vi "Global LV.vi"() -> ()   [LabVIEW 2023, in "GUI.lvlib"]
uses:
  GUI.lvlib
panel:
  out "Uniquestepld & Result Status":variant
  in  "TestCase Status":string[](array[string])
  in  "Fail Count":i32
  in  "Pass Count":i32
  out "Interlock Started?":bool
  in  "TestCase":string[](array[string])
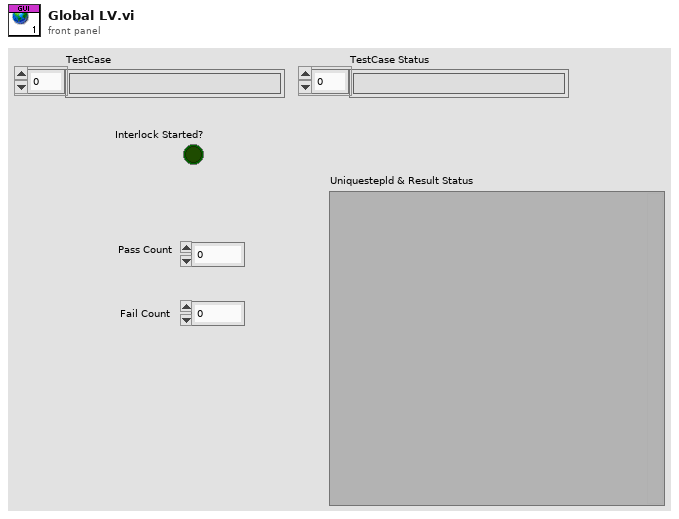
[diagram p1: front panel]
diagram:
